vi "sub init menu.vi"(8 "error in (no error)":errorcluster, 11 "IDE simple in":refnum<class "LF2R IDE.lvclass">) -> (0 "error out":errorcluster, 3 "IDE simple out":refnum<class "LF2R IDE.lvclass">)   [LabVIEW 2018, in "LF2R IDE.lvlib" / "LF2R IDE.lvclass"]
uses:
  LF2R IDE.lvclass
  Menu item.ctl
  LF2R IDE.lvclass/LF2R IDE.ctl
  <userlib>/_MGI/Menu Building/MenuItem/MenuSeparatorItem/MGI_MenuSeparatorItem.lvclass
  C:/Program Files (x86)/National Instruments/LabVIEW 2018/user.lib/_MGI/Menu Building/MenuItem/MGI_MenuItem.lvclass
  <userlib>/_MGI/Menu Building/MenuItem/MenuItem.vi
  <userlib>/_MGI/Menu Building/MenuItem/MenuSeparatorItem/MenuSeparatorItem.vi
  <userlib>/_MGI/Menu Building/MenuItem/Write Sub-Menus.vi
  <userlib>/_MGI/Menu Building/MenuTypes/Vi/VI.vi
  <userlib>/_MGI/Menu Building/MenuTypes/Vi/MGI_VI.lvclass
  <userlib>/_MGI/Menu Building/MenuTypes/MGI_Menu.lvclass
  <userlib>/_MGI/Menu Building/MenuItem/MGI_MenuItem.lvclass
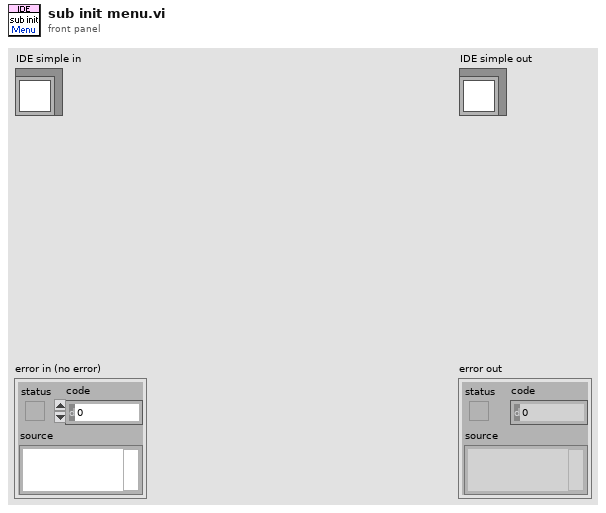
[diagram p1: front panel]
types:
  T1 = typedef "LF2R IDE.lvlib/LF2R IDE.lvclass/Menu item.ctl" = enum16{"INVALID ITEM", "Open File", "Save File", "Exit"}
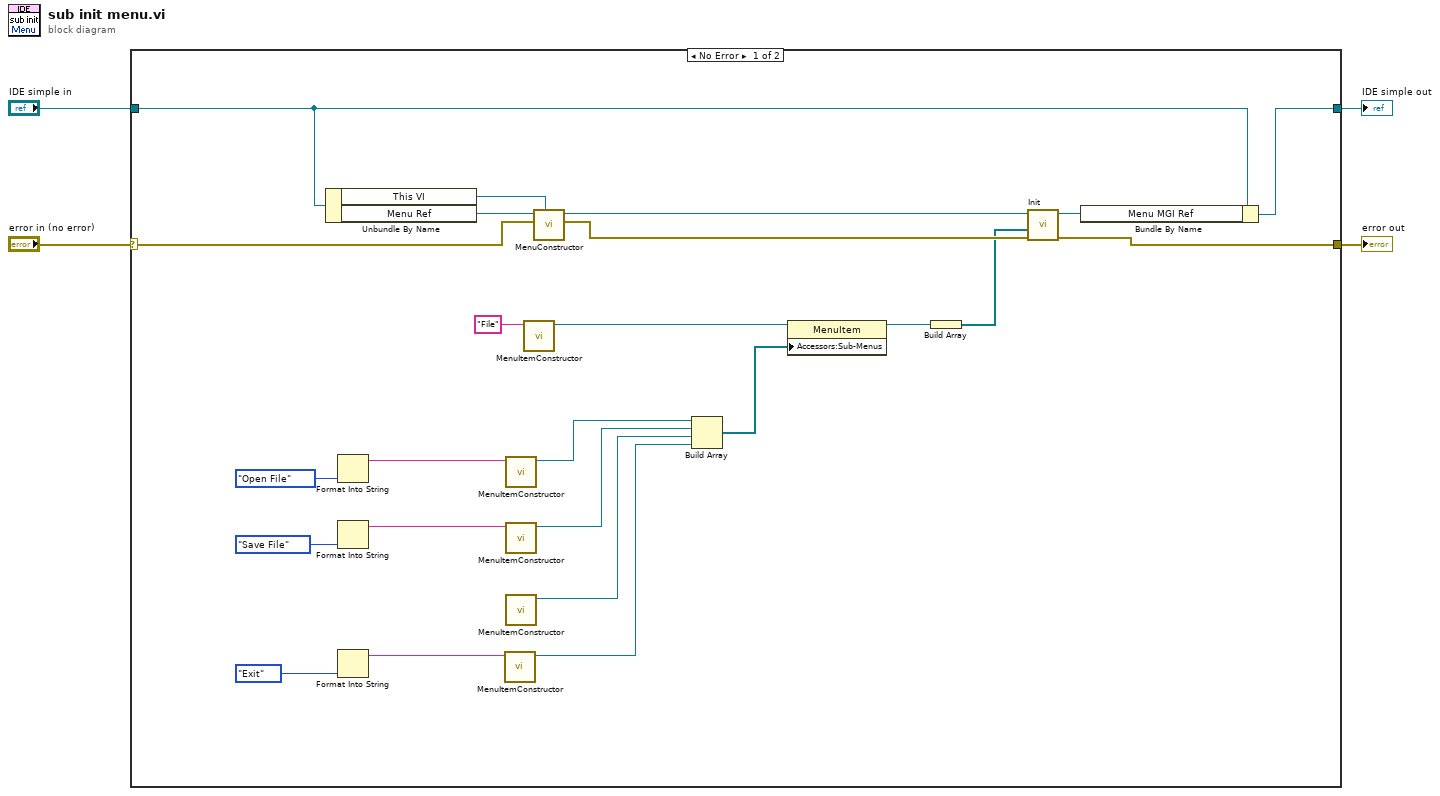
[diagram p0: block diagram]
diagram:
  n1 = case shown="No Error" "error in (no error)" {
    selector: "error in (no error)" -> [w25 w30]
    tunnel: [w5 w30] -> w3
    tunnel: [w23 w29] -> w1
    tunnel: "IDE simple in" -> [w26 w29]
    frame No Error {
      n2 = Unbundle By Name(w26) -> ("This VI"=w27:refnum<vi>, "Menu Ref"=w28:refnum<k9>)
      n3 = Format Into String(Menu_item."Open File" ("Menu item")) -> (resulting string=w13:string)  [unwired: 3 in, 1 out]
      n4 = Format Into String(Menu_item."Save File" ("Menu item")) -> (resulting string=w10:string)  [unwired: 3 in, 1 out]
      n5 = Format Into String(Menu_item."Exit" ("Menu item")) -> (resulting string=w11:string)  [unwired: 3 in, 1 out]
      n6 = call-poly <userlib>:"MenuItemConstructor.vi"("Text"=w11) -> ("MenuItem"=w18:refnum<data-value>)  [unwired: 9 in, 1 out]
      n7 = call-poly <userlib>:"MenuItemConstructor.vi"("Text"=w13) -> ("MenuItem"=w20:refnum<data-value>)  [unwired: 9 in, 1 out]
      n8 = call-poly <userlib>:"MenuItemConstructor.vi"("Text"=w10) -> ("MenuItem"=w8:refnum<data-value>)  [unwired: 9 in, 1 out]
      n9 = call-poly <userlib>:"MenuItemConstructor.vi"() -> ("MenuSeparatorItem"=w19:refnum<data-value>)  [unwired: 10 in, 1 out]
      n10 = call-poly <userlib>:"MenuItemConstructor.vi"("Text"="File") -> ("MenuItem"=w22:refnum<data-value>)  [unwired: 9 in, 1 out]
      n11 = call-poly <userlib>:"MenuConstructor.vi"("Menu VI"=w27, "error in (no error)"=w25, "menu reference"=w28) -> ("error out"=w24:errorcluster, "VI"=w7:refnum<class "MGI_VI.lvclass">)  [unwired: 7 in]
      n12 = Build Array(w20, w8, w19, w18) -> (w17:refnum<data-value>[])
      n13 = property class="MenuItem"(reference=w22, "Accessors:Sub-Menus"=w17) -> (reference out=w16:refnum<data-value>)  [unwired: 1 in, 1 out]
      n14 = Build Array(w16) -> (w15:refnum<data-value>[])
      n15 = call-dynamic "Init.vi"("error in (no error)"=w24, "Menu Items"=w15, "Menu in"=w7) -> ("error out"=w5:errorcluster, "Menu out"=w6:refnum<class "MGI_VI.lvclass">)  [unwired: 6 in, 1 out]
      n16 = Bundle By Name(cluster=w26, "Menu MGI Ref"=w6) -> (w23:refnum<class "LF2R IDE.lvclass">)
    }
    frame Error {
    }
  }
  "error out" <- w3
  "IDE simple out" <- w1
